vi "Start.vi"(8 "error in (no error)":errorcluster, 10 "Message in":refnum<class "StartMessage.lvclass">, 11 "ExampleClassC in":refnum<class "ExampleClassC.lvclass">) -> (0 "error out":errorcluster, 3 "ExampleClassC out":refnum<class "ExampleClassC.lvclass">)   [LabVIEW 2012, in "ExampleClassC.lvclass"]
doc: "This member function is called when the statemachine in the run.vi receives an 'start' command. It relays the message to all observers of the component.\n\nOverride this member function in your derived class if you need additional start functionality (but don't forget to call the parent method)."
uses:
  ExampleClassC.lvclass
  <vilib>/Distrio/Murmex/StartMessage/StartMessage.lvclass
  <vilib>/Distrio/Murmex/Murmex/Murmex.lvclass
  <vilib>/Distrio/Murmex/Message/Message.lvclass
panel:
  # "This member function is called when the statemachine in the run.vi receives an 'start' command. It relays the message to all observers of the component.\n\nOverride this member function in your derived class if you need additional start functionality (but don't forget to call the parent method)."
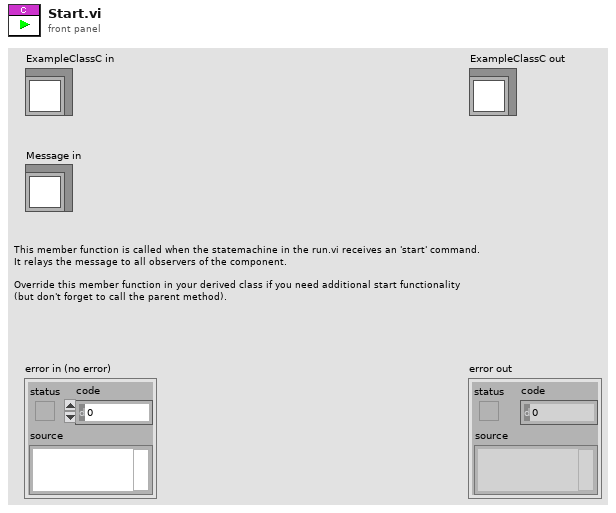
[diagram p1: front panel]
types:
  T1 = typedef "Image Type" = u32
  T2 = typedef "IMAQ Image.ctl" = refnum<image>
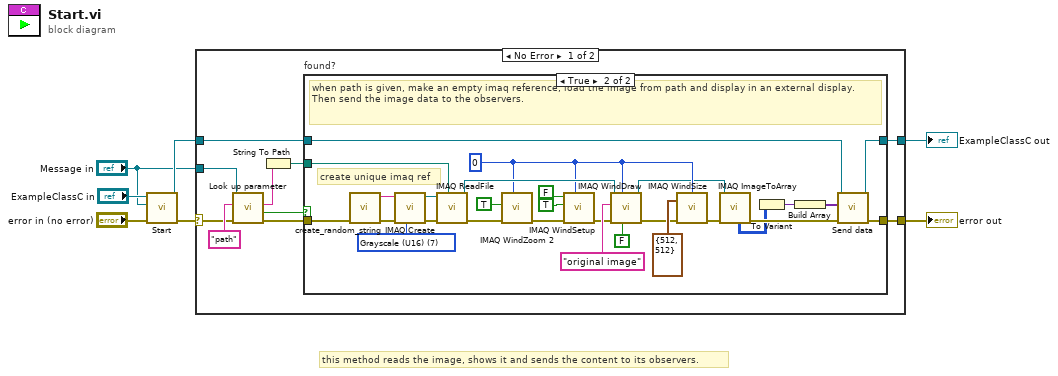
[diagram p0: block diagram]
diagram:
  # "this method reads the image, shows it and sends the content to its observers."
  n1 = call-parent "Start.vi"("error in (no error)"="error in (no error)", "Message in"="Message in", "Murmex in"="ExampleClassC in") -> ("error out"=w5:errorcluster, "Murmex out"=w2:refnum<class "ExampleClassC.lvclass">)  [unwired: 7 in]
  n2 = case shown="No Error" w5 {
    selector: w5 -> [w13 w49]
    tunnel: [w11 w49] -> w4
    tunnel: [w9 w48] -> w3
    tunnel: w2 -> [w10 w48]
    tunnel: "Message in" -> [w12 _]
    frame No Error {
      n3 = call <vilib>:"Look up parameter.vi"("error in (no error)"=w13, "name"="path", "Message in"=w12) -> ("error out"=w14:errorcluster, "found?"=w8:bool, "key"=w16:string)  [unwired: 5 in, 1 out]
      n4 = String To Path(string=w16) -> (path=w15:path)
      n5 = case "found?" shown="True" w8 {
        tunnel: w15 -> [_ w47]
        tunnel: w14 -> [w19 w21]
        tunnel: [w19 w29] -> w11
        tunnel: w10 -> [w18 w28]
        tunnel: [w18 w27] -> w9
        frame False {
          # "path missing"
        }
        frame True {
          w37 = 0 ("Window Number (0...15)")
          w44 = T1 7 items=["Grayscale (U8)", "Grayscale (I16)", "Grayscale (SGL)", "Complex (CSG)", "RGB (U32)", "HSL (U32)", "RGB (U64)", "Grayscale (U16)"] ("Image Type")
          # "create unique imaq ref"
          # "when path is given, make an empty imaq reference, load the image from path and display in an external display. Then send the image data to the observers."
          n6 = call <vilib>:"create_random_string.vi"("error in (no error)"=w21) -> ("error out"=w20:errorcluster, "random string"=w22:string)  [unwired: 9 in]
          n7 = call "IMAQ Create"("Image Name"=w22, "Image Type"=w44, "error in (no error)"=w20) -> ("New Image"=w46:T2, "error out"=w45:errorcluster)  [unwired: 2 in]
          n8 = call "IMAQ ReadFile"("File Path"=w47, "error in (no error)"=w45, "Image"=w46) -> ("error out"=w33:errorcluster, "Image Out"=w43:T2)  [unwired: 4 in, 3 out]
          n9 = call "IMAQ WindZoom 2"("Window Number (0...15)"=w37, "error in (no error)"=w33, "Zoom to Fit? (False)"=TRUE) -> ("error out"=w36:errorcluster)  [unwired: 5 in, 3 out]
          n10 = call "IMAQ WindSetup"("Window Number (0...15)"=w37, "error in (no error)"=w36, "Window can close? (Yes)"=TRUE, "Window can grow? (Yes)"=FALSE) -> ("error out"=w35:errorcluster)  [unwired: 7 in]
          n11 = call "IMAQ WindDraw"("Resize to Image Size? (Y)"=FALSE, "Window Number (0...15)"=w37, "error in (no error)"=w35, "Title"="original image", "Image"=w43) -> ("error out"=w34:errorcluster, "Image Out (duplicate)"=w30:T2)  [unwired: 5 in]
          n12 = call "IMAQ WindSize"("error in (no error)"=w34, "Width & Height"=cluster{"Width":i32, "Height":i32} {"Width"=512, "Height"=512}, "Window Number"=w37) -> ("error out"=w32:errorcluster)  [unwired: 3 in, 2 out]
          n13 = call "IMAQ ImageToArray"("error in (no error)"=w32, "Image"=w30) -> ("Image Pixels (U16)"=w26:u16[][], "error out"=w31:errorcluster)  [unwired: 2 in, 3 out]
          n14 = To Variant(anything=w26) -> (Variant=w25:variant)
          n15 = Build Array(w25) -> (w24:variant[])
          n16 = call <vilib>:"Send data.vi"("error in (no error)"=w31, "data (channels array)"=w24, "Murmex in"=w28) -> ("error out"=w29:errorcluster, "Murmex out"=w27:refnum<class "ExampleClassC.lvclass">)  [unwired: 7 in]
        }
      }
    }
    frame Error {
    }
  }
  "error out" <- w4
  "ExampleClassC out" <- w3
